vi "FTW-JSON-Object-GetElement-DBL.vi"(0 "JSON Object":refnum<data-value>, 5 "Key":string, 7 "Default Value":dbl=nan, 11 "error in":errorcluster) -> (4 "JSON Object out":refnum<data-value>, 8 "Value":dbl, 10 "Found?":bool, 15 "error out":errorcluster)   [LabVIEW 2014]
uses:
  core/FTW-JSON-Core-Structure.ctl
  error/FTW-ERR-ThrowGenericError.vi
  error/FTW-ERR-ThrowError.vi
  error/FTW-ERR-NoErrorConstant.vi
  error/FTW-ERR-CallChain.vi
  string/FTW-STR-ReplaceWhitespace.vi
panel:
  # "Inputs"
  # "Outputs"
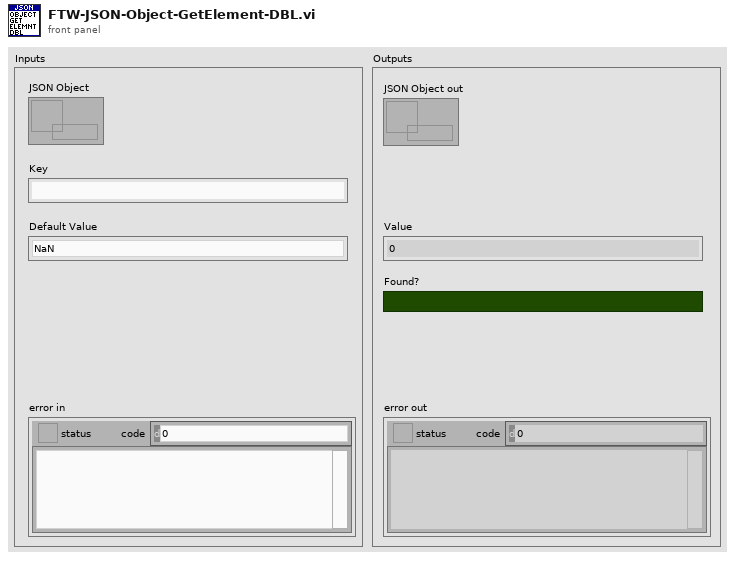
[diagram p1: front panel]
types:
  T1 = typedef "FTW-JSON-Core-Structure.ctl" = cluster{"JSON Object":i64, "Encoding Flags":i64, "Decoding Flags":i64}
  T2 = typedef "FTW-JSON-Core-Type.ctl" = enum16{"Object", "Array", "String", "Integer", "Floating Point", "true", "false", "null", "undefined"}
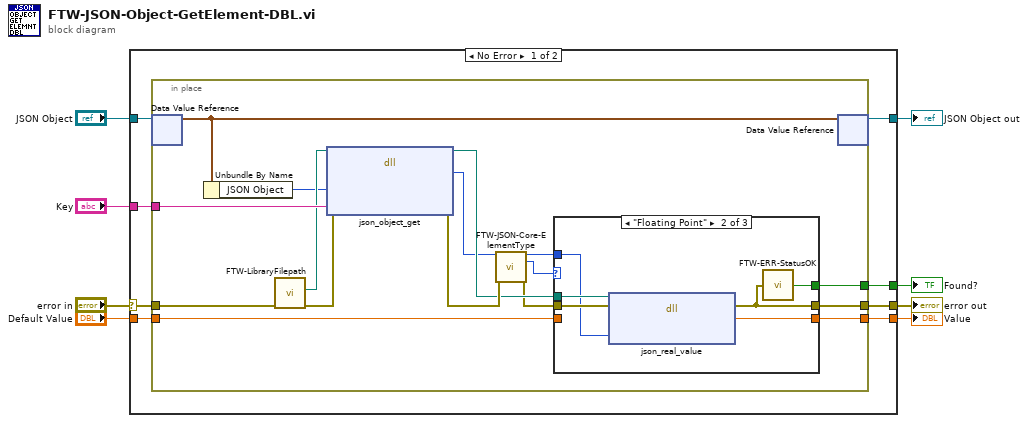
[diagram p0: block diagram]
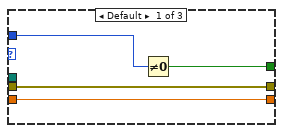
[diagram p2: hidden frame]
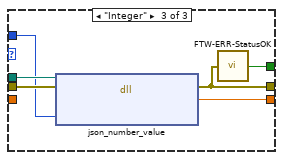
[diagram p3: hidden frame]
diagram:
  n1 = case shown="No Error" "error in" {
    selector: "error in" -> [w16 w51]
    tunnel: [w14 w51] -> w8
    tunnel: [w9 w50] -> w6
    tunnel: "JSON Object" -> [w10 w50]
    tunnel: "Key" -> [w15 _]
    tunnel: [w13 w49] -> w3
    tunnel: [w12 _] -> w2
    tunnel: "Default Value" -> [w11 w49]
    frame No Error {
      n2 = in-place {
        in-place-border: w16 -> [w32]
        in-place-border: w15 -> [w31]
        in-place-border: [w27] -> w14
        in-place-border: [w26] -> w13
        in-place-border: [w24] -> w12
        in-place-border: w11 -> [w19]
        n3 = in-place-dvr #1(w10) -> (w18:T1)  [unwired: 1 out]
        n4 = Unbundle By Name(w18) -> ("JSON Object"=w17:i64)
        n5 = call "FTW-LibraryFilepath.vi"("error in"=w32) -> ("error out"=w30:errorcluster, "Library Filepath"=w29:path)  [unwired: 8 in, 1 out]
        n6 = dll-call lib="?" fn="json_object_get"(path in=w29, error in=w30, "JSON Object Pointer"=w17, "Element Key"=w31) -> (path out=w25:path, error out=w28:errorcluster, "JSON Element Pointer"=w22:i64)  [unwired: 3 in]
        n7 = call "FTW-JSON-Core-ElementType.vi"("JSON Element"=w22, "error in"=w28) -> ("JSON Element out"=w21:i64, "JSON Type"=w20:T2, "error out"=w23:errorcluster)  [unwired: 11 in]
        n8 = case shown="\"Floating Point\"" w20 {
          tunnel: [w36 w42 w48] -> w27
          tunnel: [w33 w41 w47] -> w26
          tunnel: w25 -> [_ w40 w46]
          tunnel: [w34 w39 w45] -> w24
          tunnel: w23 -> [w36 w38 w44]
          tunnel: w21 -> [w35 w37 w43]
          tunnel: w19 -> [w33 _ _]
          frame Default {
            n9 = Not Equal To 0?(x=w35) -> (x != 0?=w34:bool)
          }
          frame "Floating Point" {
            n10 = dll-call lib="?" fn="json_real_value"(path in=w40, error in=w38, "JSON Element Pointer"=w37) -> (error out=w42:errorcluster, "DBL Value"=w41:dbl)  [unwired: 2 in, 1 out]
            n11 = call "FTW-ERR-StatusOK.vi"("error to check"=w42) -> ("Status OK?"=w39:bool)
          }
          frame "Integer" {
            n12 = dll-call lib="?" fn="json_number_value"(path in=w46, error in=w44, "JSON Element Pointer"=w43) -> (error out=w48:errorcluster, "DBL Value"=w47:dbl)  [unwired: 2 in, 1 out]
            n13 = call "FTW-ERR-StatusOK.vi"("error to check"=w48) -> ("Status OK?"=w45:bool)
          }
        }
        n14 = in-place-dvr #1(w18) -> (w9:refnum<data-value>)  [unwired: 1 out]
      }
    }
    frame Error {
    }
  }
  "error out" <- w8
  "JSON Object out" <- w6
  "Value" <- w3
  "Found?" <- w2
